vi "Propagate Error.vi"(8 "error in":errorcluster, 10 "Issued VI":refnum<vi>, 11 "queue out":refnum<queue>) -> (0 "error out":errorcluster)   [LabVIEW 2024, in "Error Handler.lvlib"]
uses:
  Error Handler.lvlib
  Support/General Type Defs/Queue Message.ctl
  Support/General Type Defs/General Type Definitions.lvlib
  Support/General Type Defs/Error Handler Data.ctl
  Error Queue - Enqueue.vi
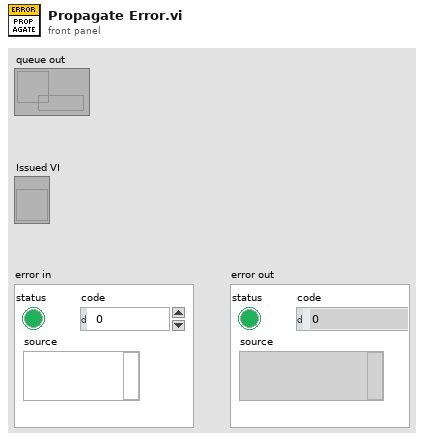
[diagram p1: front panel]
types:
  T1 = typedef "General Type Definitions.lvlib/Error Handler Data.ctl" = cluster{"Module":string, "Error Data":errorcluster, "Last Queue Message":T2}
  T2 = typedef "General Type Definitions.lvlib/Queue Message.ctl" = cluster{"Message":string, "Value":variant}
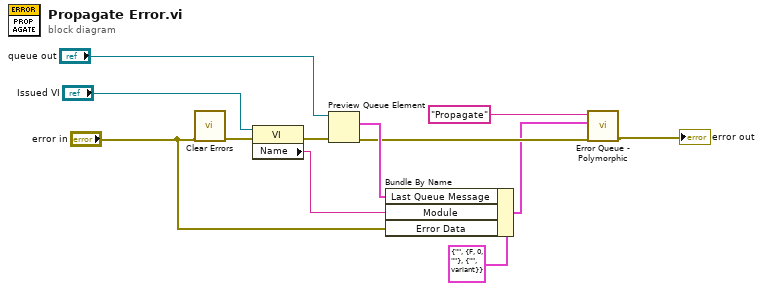
[diagram p0: block diagram]
diagram:
  n1 = call <vilib>:"Clear Errors.vi"("error in (no error)"="error in") -> ("error out"=w11:errorcluster)  [unwired: 5 in, 1 out]
  n2 = property class="VI"(reference="Issued VI", error in=w11) -> (error out=w9:errorcluster, "Name"=w6:string)  [unwired: 1 out]
  n3 = Preview Queue Element(queue="queue out", error in (no error)=w9) -> (element=w7:T2, error out=w4:errorcluster)  [unwired: 1 in, 2 out]
  n4 = Bundle By Name(cluster=T1 {"Module"="", "Error Data"={"status"=FALSE, "code"=0, "source"=""}, "Last Queue Message"={"Message"="", "Value"=variant}} ("Error Handler Data"), "Last Queue Message"=w7, "Module"=w6, "Error Data"="error in") -> (w3:T1)
  n5 = call-poly "Error Queue - Polymorphic.vi"("error in"=w4, "Value"=w3, "Message"="Propagate") -> ("error out"=→"error out":errorcluster)  [unwired: 8 in]
